vi "Read Front Tunnel Internal TermRefs.vi"(8 "error in (no error)":errorcluster, 10 "case":string, 11 "CSM-Helper in":refnum<class "CSM-Helper.lvclass">) -> (0 "error out":errorcluster, 2 "Front Tunnels":T1, 3 "CSM-Helper out":refnum<class "CSM-Helper.lvclass">)   [LabVIEW 2020, in "CSM-Helper.lvclass"]
uses:
  CSM-Helper.lvclass
  CSM-Helper.lvclass/CSM-Helper.ctl
  Read Front Tunnels Refs.vi
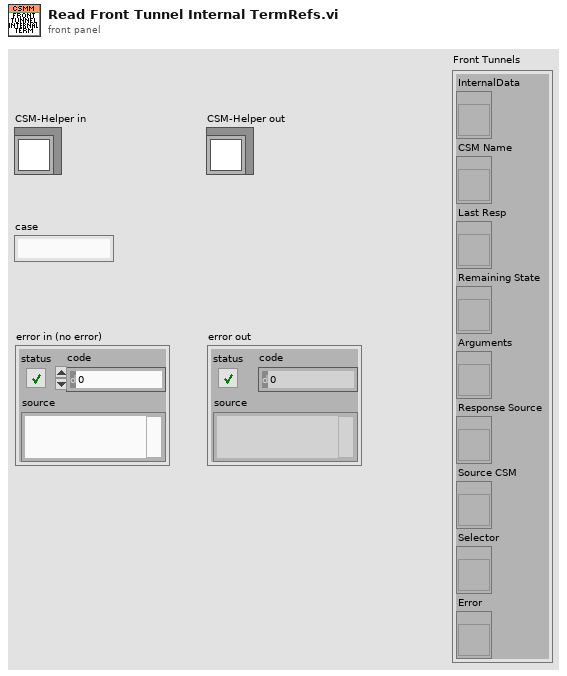
[diagram p1: front panel]
types:
  T1 = cluster{"InternalData":refnum<vi>, "CSM Name":refnum<vi>, "Last Resp":refnum<vi>, "Remaining State":refnum<vi>, "Arguments":refnum<vi>, "Response Source":refnum<vi>, "Source CSM":refnum<vi>, "Selector":refnum<vi>, "Error":refnum<vi>}
  T2 = typedef "CSM-Helper.lvclass/_csmhelper_Front_Tunnels_Refs.ctl" = cluster{"InternalData":refnum<vi>, "CSM Name":refnum<vi>, "Last Resp":refnum<vi>, "Remaining State":refnum<vi>, "Arguments":refnum<vi>, "Response Source":refnum<vi>, "Source CSM":refnum<vi>, "Selector":refnum<vi>, "Error":refnum<vi>}
  T3 = cluster{refnum<vi>, refnum<vi>, refnum<vi>, refnum<vi>, refnum<vi>, refnum<vi>, refnum<vi>, refnum<vi>, refnum<vi>}
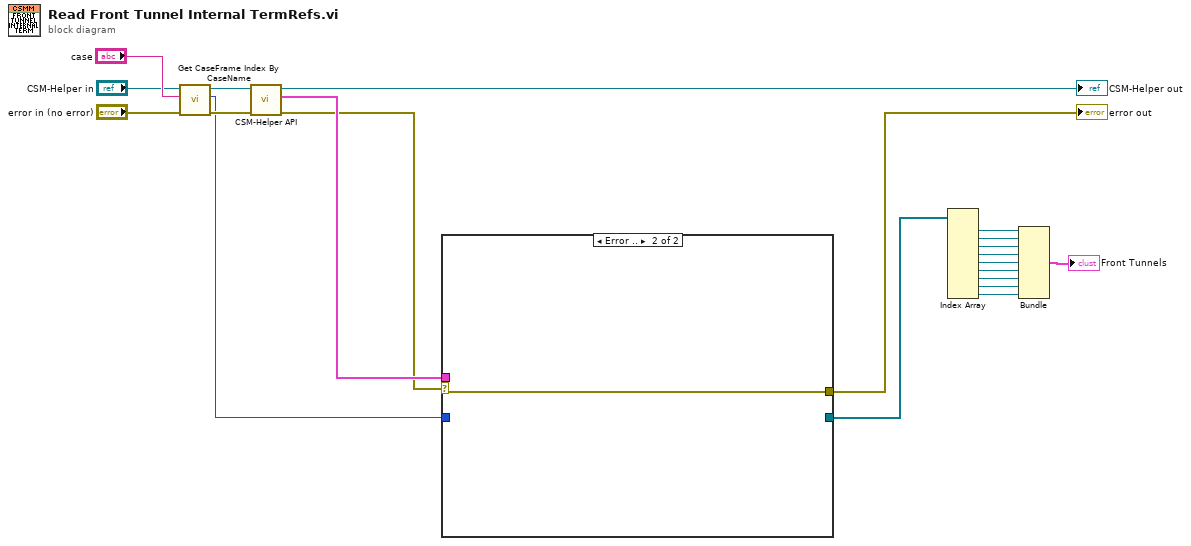
[diagram p0: block diagram]
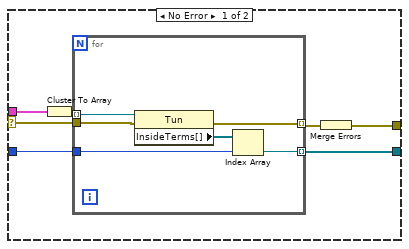
[diagram p2: hidden frame]
diagram:
  n1 = call "Get CaseFrame Index By CaseName.vi"("error in (no error)"="error in (no error)", "CASE"="case", "CSM-Helper in"="CSM-Helper in") -> ("error out"=w20:errorcluster, "index"=w14:i32, "CSM-Helper out"=w18:refnum<class "CSM-Helper.lvclass">)  [unwired: 6 in]
  n2 = call-poly "CSM-Helper API.vi"("error in (no error)"=w20, "CSM-Helper in"=w18) -> ("error out"=w12:errorcluster, "Front Tunnels"=w21:T2, "CSM-Helper out"=→"CSM-Helper out":refnum<class "CSM-Helper.lvclass">)  [unwired: 7 in]
  n3 = case shown="Error .." w12 {
    selector: w12 -> [w23 w35]
    tunnel: w21 -> [w28 _]
    tunnel: w14 -> [w27 _]
    tunnel: [w26 _] -> w13
    tunnel: [w22 w35] -> w11
    frame No Error {
      n4 = Cluster To Array(cluster=w28) -> (array=w25:refnum<vi>[])
      n5 = for {
        tunnel: w27 -> [w33]
        tunnel: [w32] -> w26 mode=indexing
        tunnel: w25 -> [w31] mode=indexing
        tunnel: w23 -> [w30]
        tunnel: [w29] -> w24 mode=indexing
        n6 = property on="Property Node" class="Tun"(reference=w31, error in=w30) -> (error out=w29:errorcluster, "InsideTerms[]"=w34:refnum<vi>[])  [unwired: 1 out]
        n7 = Index Array(array=w34, index=w33) -> (element=w32:refnum<vi>)
      }
      n8 = Merge Errors(w24) -> (w22:errorcluster)
    }
    frame Error {
    }
  }
  "error out" <- w11
  n9 = Index Array(array=w13) -> (element #1=w10:refnum<vi>, element #2=w9:refnum<vi>, element #3=w8:refnum<vi>, element #4=w7:refnum<vi>, element #5=w6:refnum<vi>, element #6=w5:refnum<vi>, element #7=w4:refnum<vi>, element #8=w3:refnum<vi>, element #9=w2:refnum<vi>)  [unwired: 9 in]
  n10 = Bundle(w10, w9, w8, w7, w6, w5, w4, w3, w2) -> (→"Front Tunnels":T3)  [unwired: 1 in]
